vi "读取数据库.vi"(5 "精度(6)":i16=2, 7 "condition":string, 8 "error in (no error)":errorcluster caption="错误输入（无错误）", 9 "database":string="database1.mdb", 10 "显示项":string[](array[string]), 11 "组合框":string(combo)) -> (0 "error out":errorcluster caption="错误输出", 1 "columns":string[](array[string]), 2 "data":variant[][](array[variant]), 3 "表格":string[][](table))   [LabVIEW 2016]
uses:
  <vilib>/Utility/sysdir.llb/System Directory Type.ctl
  <vilib>/addons/database/Connection.llb/DB Tools Open Connec (String).vi
  <vilib>/addons/database/_DB Variant To Data/Database Variant To Data.xnode
  <vilib>/addons/database/NI_Database_API.lvlib
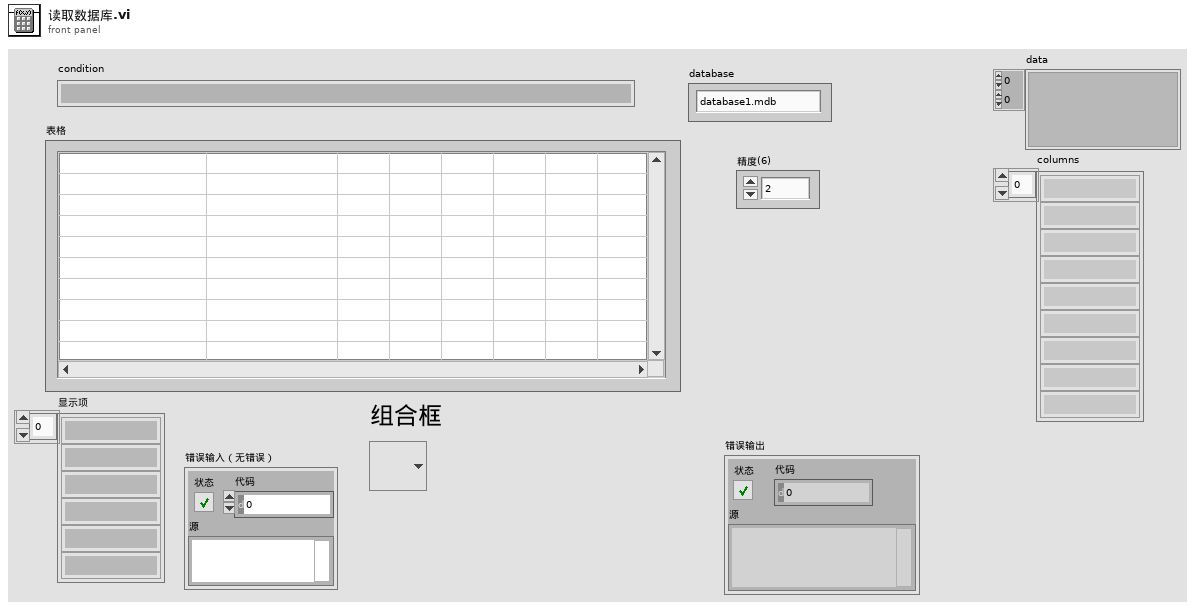
[diagram p1: front panel]
types:
  T1 = typedef "System Directory Type.ctl" = i32
  T2 = typedef "NI_Database_API.lvlib/Conn ObjectReference.ctl" = refnum<k1>
  T3 = typedef "NI_Database_API.lvlib/DB Tools DataTypes.ctl" = enum16{"String", "Long (I32)", "Single (SGL)", "Double (DBL)", "Date/Time", "Binary"}
  T4 = cluster{"name":string, "database data type":T3, "defined size":i32}[]
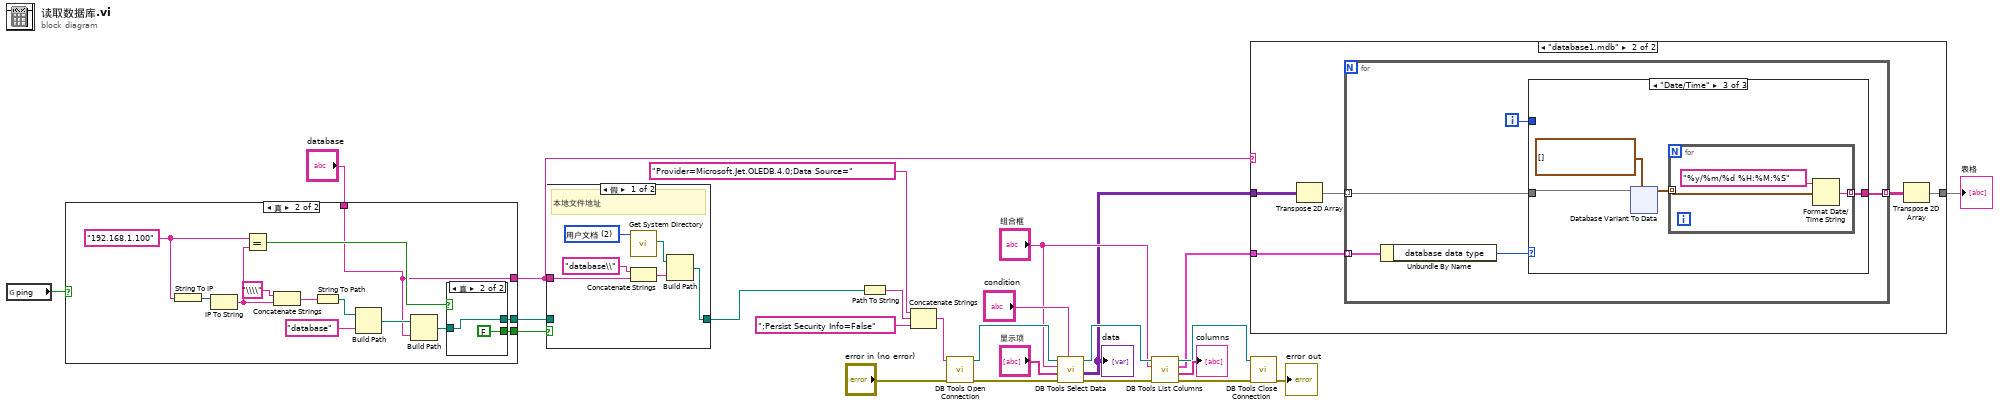
[diagram p0: block diagram]
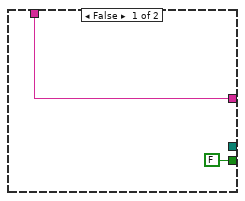
[diagram p2: hidden frame]
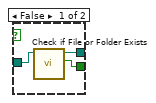
[diagram p3: hidden frame]
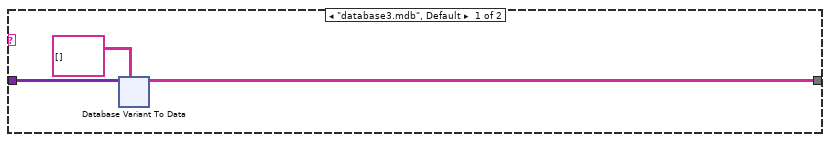
[diagram p5: hidden frame]
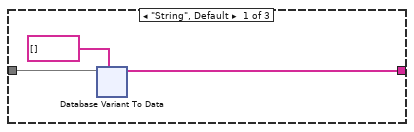
[diagram p6: hidden frame]
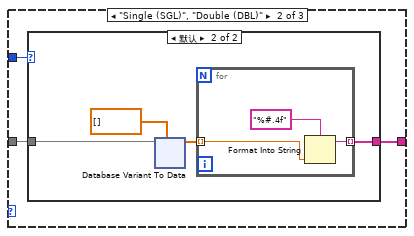
[diagram p7: hidden frame]
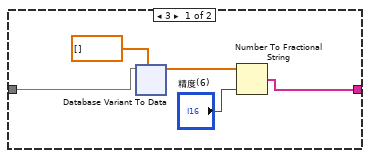
[diagram p8: hidden frame]
diagram:
  n1 = global read "ping全局.vi" "ping"() -> (w2:bool)
  n2 = case shown="真" w2 {
    tunnel: [_ w31] -> w6
    tunnel: [FALSE ("file or folder exists?") w30] -> w5
    tunnel: [w26 w28] -> w3
    tunnel: "database" -> [w26 w28]
    frame False {
    }
    frame True {
      w29 = "192.168.1.100" ("名称")
      n3 = String To IP(1:w29) -> (0:w40:u32)
      n4 = IP To String(2:w40) -> (0:w34:string)  [unwired: 1 in]
      n5 = Equal?(x=w29, y=w34) -> (x = y?=w33:bool)
      n6 = Concatenate Strings("\\\\" ("字符串"), w34) -> (w37:string)
      n7 = String To Path(string=w37) -> (path=w39:path)
      n8 = Build Path(base path=w39, name or relative path="database" ("名称或相对路径")) -> (appended path=w35:path)
      n9 = Build Path(base path=w35, name or relative path=w28) -> (appended path=w32:path)
      n10 = case shown="真" w33 {
        tunnel: w32 -> [w43 w44]
        tunnel: [w42 w44] -> w31
        tunnel: [w41 FALSE] -> w30
        frame False {
          n11 = call <vilib>:"Check if File or Folder Exists.vi"("path"=w43) -> ("file or folder exists?"=w41:bool, "dup path"=w42:path)  [unwired: 8 in, 1 out]
        }
        frame True {
        }
      }
    }
  }
  n12 = case shown="假" w5 {
    tunnel: w3 -> [w47 _]
    tunnel: w6 -> [_ w52]
    tunnel: [w46 w52] -> w4
    frame False {
      w51 = T1 2 items=["用户目录"=0, "用户桌面"=1, "用户文档"=2, "用户应用程序数据"=3, "用户设置"=4, "用户临时目录"=5, "公共文档"=6, "公共应用程序数据"=7, "公共设置"=8, "公共缓存"=13, "系统核心库"=9, "系统安装库"=10, "应用程序文件"=11, "启动盘根目录"=12] ("system directory type")
      # "本地文件地址"
      n13 = call <vilib>:"Get System Directory.vi"("system directory type"=w51) -> ("system directory"=w50:path)  [unwired: 10 in]
      n14 = Concatenate Strings("database\\" ("名称或相对路径"), w47) -> (w48:string)
      n15 = Build Path(base path=w50, name or relative path=w48) -> (appended path=w46:path)
    }
    frame True {
      # "网络共享地址"
    }
  }
  n16 = Path To String(path=w4) -> (string=w12:string)
  n17 = Concatenate Strings("Provider=Microsoft.Jet.OLEDB.4.0;Data Source=", w12, ";Persist Security Info=False") -> (w11:string)
  n18 = call-poly <vilib>:"DB Tools Open Connection.vi"("error in (no error)"="error in (no error)", "connection information"=w11) -> ("error out"=w24:errorcluster, "connection reference"=w25:T2)  [unwired: 6 in]
  n19 = call <vilib>:"DB Tools Select Data.vi"("condition"="condition", "error in (no error)"=w24, "columns"="显示项", "table"="组合框", "connection reference"=w25) -> ("error out"=w23:errorcluster, "data"=w9:variant[][], "connection reference out"=w20:T2)  [unwired: 1 in]
  "data" <- w9
  n20 = call <vilib>:"DB Tools List Columns.vi"("error in (no error)"=w23, "table"="组合框", "connection reference"=w20) -> ("error out"=w15:errorcluster, "columns"=→"columns":string[], "column information"=w8:T4, "connection reference out"=w16:T2)  [unwired: 1 in]
  n21 = case shown="\"database1.mdb\"" w3 {
    tunnel: w9 -> [w54 w104]
    tunnel: w8 -> [_ w102]
    tunnel: [w53 w100] -> w7
    frame "database3.mdb", Default {
      n22 = xnode "Database Variant To Data"("database variant"=w54, "type"=string[][] []) -> ("data"=w53:string[][])  [unwired: 1 in, 1 out]
    }
    frame "database1.mdb" {
      n23 = Transpose 2D Array(2D array=w104) -> (transposed array=w103:variant[][])
      n24 = for {
        tunnel: w103 -> [w107] mode=indexing
        tunnel: w102 -> [w109] mode=indexing
        tunnel: [w106] -> w101 mode=indexing
        i -> [w105]
        n25 = Unbundle By Name(w109) -> ("database data type"=w108:T3)
        n26 = case shown="\"Date/Time\"" w108 {
          tunnel: w107 -> [w111 w153 w244]
          tunnel: [w110 w152 w242] -> w106
          tunnel: w105 -> [_ w151 _]
          frame "String", Default {
            n27 = xnode "Database Variant To Data"("database variant"=w111, "type"=string[] []) -> ("data"=w110:string[])  [unwired: 1 in, 1 out]
          }
          frame "Single (SGL)", "Double (DBL)" {
            n28 = case shown="默认" w151 {
              tunnel: w153 -> [w158 w199]
              tunnel: [w154 w197] -> w152
              frame 3 {
                n29 = xnode "Database Variant To Data"("database variant"=w158, "type"=dbl[] []) -> ("data"=w156:dbl[])  [unwired: 1 in, 1 out]
                n30 = Number To Fractional String(number=w156, precision (6)="精度(6)") -> (F-format string=w154:string[])  [unwired: 2 in]
              }
              frame Default {
                n31 = xnode "Database Variant To Data"("database variant"=w199, "type"=dbl[] []) -> ("data"=w198:dbl[])  [unwired: 1 in, 1 out]
                n32 = for {
                  tunnel: w198 -> [w203] mode=indexing
                  tunnel: [w201] -> w197 mode=indexing
                  n33 = Format Into String(format string="%#.4f" ("格式字符串"), w203) -> (resulting string=w201:string)  [unwired: 2 in, 1 out]
                }
              }
            }
          }
          frame "Date/Time" {
            n34 = xnode "Database Variant To Data"("database variant"=w244, "type"=timestamp[] []) -> ("data"=w243:timestamp[])  [unwired: 1 in, 1 out]
            n35 = for {
              tunnel: w243 -> [w247] mode=indexing
              tunnel: [w246] -> w242 mode=indexing
              n36 = Format Date/Time String(time format string (%c)="%y/%m/%d %H:%M:%S" ("时间格式字符串(%c)"), seconds (now)=w247) -> (date/time string=w246:string)  [unwired: 1 in]
            }
          }
        }
      }
      n37 = Transpose 2D Array(2D array=w101) -> (transposed array=w100:string[][])
    }
  }
  "表格" <- w7
  n38 = call <vilib>:"DB Tools Close Connection.vi"("error in (no error)"=w15, "connection reference"=w16) -> ("error out"=→"error out":errorcluster)  [unwired: 5 in]
